vi "Create Figures 3.1.vi"(8 "Error In":errorcluster, 11 "Data Cluster":T1={"Selected File"=path "", "Full Text File"=[], "Data Array"=[], "Times Array"=[], "Sensor Array"=[], "Subset Array"=[], "Smoothness Values"=[], "Sensor Select 1"=refnum, "Sensor Select 2"=refnum, "Sensor Select 3"=refnum, "Sensor Select 4"=refnum, "Start Times"=[], "End Times"=[], "Cursor List"=[{"Name"="Event Marker          ", "Color"=16777200, "Style"=0, "Point Style"=0, "Name Visible"=FALSE, "Allow Drag"=FALSE, "Cursor Mode"=0, "Plot"=0, "Index"=0, "Position"={"X"=4.0, "Y"=1.0}, "X Scale"=0, "Y Scale"=0, "Watch Plots"=[], "Watch All Plots"=FALSE, "Plot Area"=0, "Label Offset"={"X"=-50.0, "Y"=150.0}}, {"Name"="Upper Sensor", "Color"=13816500, "Style"=6, "Point Style"=0, "Name Visible"=FALSE, "Allow Drag"=FALSE, "Cursor Mode"=0, "Plot"=0, "Index"=0, "Position"={"X"=-1.0, "Y"=5.0}, "X Scale"=0, "Y Scale"=0, "Watch Plots"=[], "Watch All Plots"=FALSE, "Plot Area"=0, "Label Offset"={"X"=0.0, "Y"=0.0}}, {"Name"="Lower Sensor", "Color"=13816500, "Style"=6, "Point Style"=0, "Name Visible"=FALSE, "Allow Drag"=FALSE, "Cursor Mode"=0, "Plot"=0, "Index"=0, "Position"={"X"=-1.0, "Y"=30.0}, "X Scale"=0, "Y Scale"=0, "Watch Plots"=[], "Watch All Plots"=FALSE, "Plot Area"=0, "Label Offset"={"X"=0.0, "Y"=0.0}}], "Listbox 1"=refnum, "Listbox 2"=refnum, "Listbox 3"=refnum, "Listbox 4"=refnum, "Labels"=["Why", "is", "this", "still", "not", "built", "into", "Labview?", "This", "is", "shameful."], "Event Array"=[], "Event Names"=[], "Event Times"=[], "Save Plot Button"=refnum, "Sensor Plot Refs"=[], "Selected Event (Title)"="", "Upper Cursor"=0.0, "Lower Cursor"=0.0, "Z Max"=0.0, "Z Min"=0.0}) -> (0 "Error Out":errorcluster, 3 "Message":string)   [LabVIEW 2020]
uses:
  Controls/DataCluster.ctl
  <vilib>/Utility/miscctls.llb/LVCursorListTypeDef.ctl
panel:
  in  "Home Button":bool
  in  "Spatio Button":bool
  in  "Bar Plot Button":bool
  in  "Sprectral Plot Button":bool
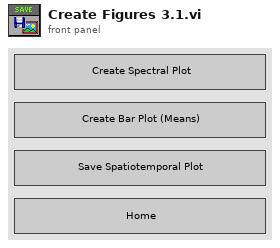
[diagram p1: front panel]
types:
  T1 = typedef "DataCluster.ctl" = cluster{"Selected File":path, "Full Text File":string[][], "Data Array":dbl[][], "Times Array":dbl[], "Sensor Array":dbl[], "Subset Array":dbl[][], "Smoothness Values":dbl[], "Sensor Select 1":refnum<vi>, "Sensor Select 2":refnum<vi>, "Sensor Select 3":refnum<vi>, "Sensor Select 4":refnum<vi>, "Start Times":dbl[], "End Times":dbl[], "Cursor List":T2, "Listbox 1":refnum<vi>, "Listbox 2":refnum<vi>, "Listbox 3":refnum<vi>, "Listbox 4":refnum<vi>, "Labels":string[], "Event Array":dbl[][], "Event Names":string[], "Event Times":dbl[], "Save Plot Button":refnum<vi>, "Sensor Plot Refs":refnum<vi>[], "Selected Event (Title)":string, "Upper Cursor":dbl, "Lower Cursor":dbl, "Z Max":dbl, "Z Min":dbl}
  T2 = typedef "LVCursorListTypeDef.ctl" = cluster{"Name":string, "Color":u32, "Style":u8, "Point Style":u8, "Name Visible":bool, "Allow Drag":bool, "Cursor Mode":u32, "Plot":i32, "Index":i32, "Position":cluster{"X":dbl, "Y":dbl}, "X Scale":u32, "Y Scale":u32, "Watch Plots":i32[], "Watch All Plots":bool, "Plot Area":i32, "Label Offset":cluster{"X":dbl, "Y":dbl}}[]
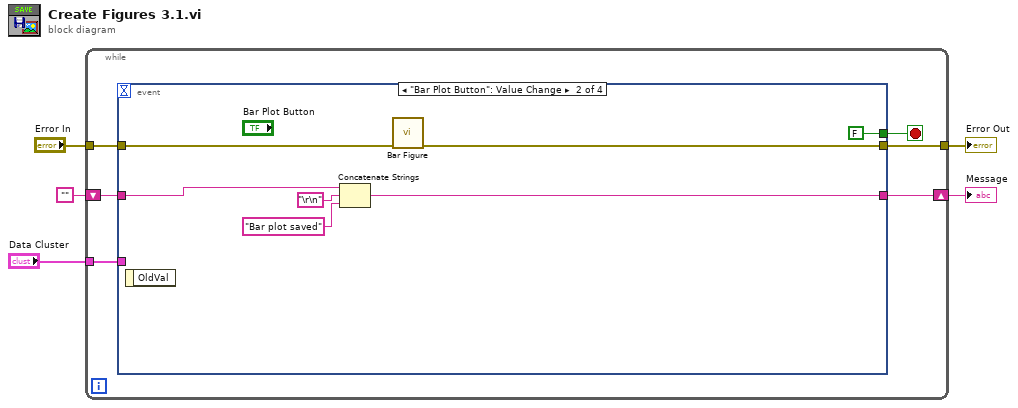
[diagram p0: block diagram]
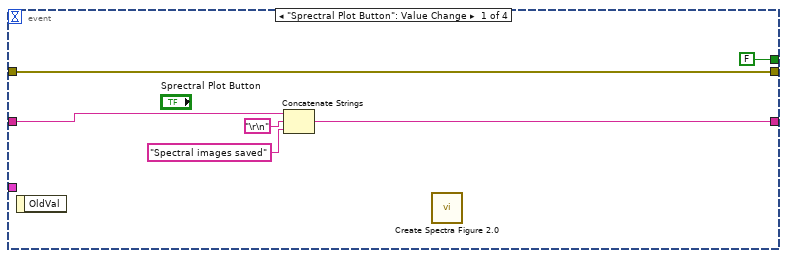
[diagram p2: hidden frame]
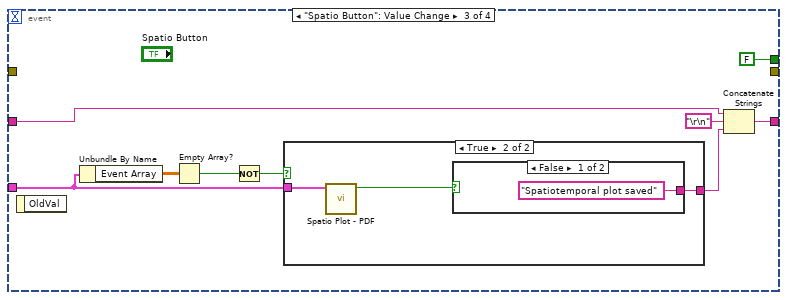
[diagram p3: hidden frame]
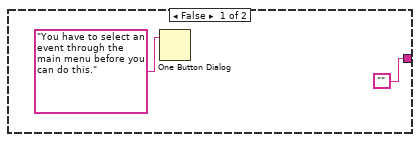
[diagram p4: hidden frame]
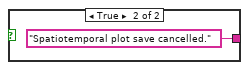
[diagram p5: hidden frame]
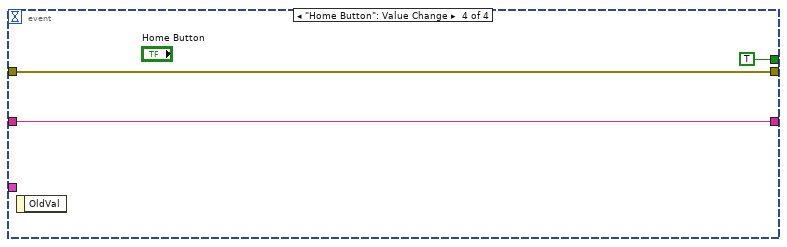
[diagram p6: hidden frame]
diagram:
  n1 = while {
    tunnel: "Error In" -> [w10]
    tunnel: "Data Cluster" -> [w9]
    tunnel: [w7] -> w3
    shift-right: [w8] -> w4
    shift-left: "" -> [w6]
    stop <- w11 stop-if-true
    n2 = event shown="[1] \"Bar Plot Button\": Value Change" {
      selector: _ -> [_ _ _ _]
      dyn-events: _ -> [_ _ _ _]
      timeout: _ -> [_ _ _ _]
      tunnel: [FALSE FALSE FALSE TRUE] -> w11
      tunnel: w10 -> [w12 w19 _ w41]
      tunnel: w9 -> [_ _ w27 _]
      tunnel: [w16 w23 w30 w42] -> w8
      tunnel: [w12 w18 _ w41] -> w7
      tunnel: w6 -> [w14 w22 w31 w42]
      event "Sprectral Plot Button": Value Change {
        n3 = event-data() -> ()  [unwired: 1 in, 1 out]
        n4 = Concatenate Strings(w14, "\r\n", "Spectral images saved" ("string")) -> (w16:string)
        n5 = call "Create Spectra Figure 2.0.vi"() -> ()  [unwired: 12 in]
      }
      event "Bar Plot Button": Value Change {
        n6 = event-data() -> ()  [unwired: 1 in, 1 out]
        n7 = Concatenate Strings(w22, "\r\n", "Bar plot saved" ("string")) -> (w23:string)
        n8 = call "Bar Figure.vi"("error in"=w19) -> ("error out"=w18:errorcluster)  [unwired: 10 in]
      }
      event "Spatio Button": Value Change {
        # "Pulls the data for the selected segment from the Data Cluster and plots it in a hidden graph. The graph is then saved as a PNG"
        n9 = event-data() -> ()  [unwired: 1 in, 1 out]
        n10 = Unbundle By Name(w27) -> ("Event Array"=w28:dbl[][])
        n11 = Empty Array?(array=w28) -> (empty?=w29:bool)
        n12 = Not(x=w29) -> (.not. x?=w26:bool)
        n13 = case shown="True" w26 {
          tunnel: w27 -> [_ w38]
          tunnel: ["" w36] -> w25
          frame False {
            n14 = One Button Dialog(message="You have to select an event through the main menu before you can do this.") -> ()  [unwired: 1 in, 1 out]
          }
          frame True {
            n15 = call "Spatio Plot - PDF.vi"("Data Cluster"=w38) -> ("cancelled"=w37:bool)  [unwired: 10 in]
            n16 = case shown="False" w37 {
              tunnel: ["Spatiotemporal plot saved" ("string") "Spatiotemporal plot save cancelled." ("string")] -> w36
              frame False {
              }
              frame True {
              }
            }
          }
        }
        n17 = Concatenate Strings(w31, "\r\n", w25) -> (w30:string)
      }
      event "Home Button": Value Change {
        n18 = event-data() -> ()  [unwired: 1 in, 1 out]
      }
    }
  }
  "Error Out" <- w3
  "Message" <- w4
